vi "Setup.vi"(10 "Queue Actor":refnum<class "Queue Actor.lvclass">, 11 "Queue Actor in":refnum<class "Queue Actor.lvclass">) -> (3 "Queue Actor out":refnum<class "Queue Actor.lvclass">)   [LabVIEW 2021, in "Queue Actor.lvclass"]
uses:
  Queue Actor.lvclass
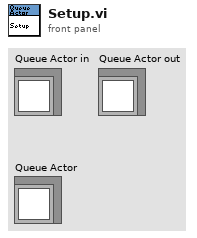
[diagram p1: front panel]
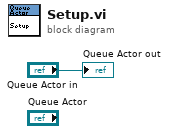
[diagram p0: block diagram]
diagram:
  "Queue Actor out" <- "Queue Actor in"
